vi "Handle.vi"(8 "error in (no error)":errorcluster, 10 "Zero Timeout Message Handler in":refnum<class "Zero Timeout Message Handler.lvclass">, 11 "Message in":refnum<class "Stop Msg.lvclass">) -> (0 "error out":errorcluster, 2 "Zero Timeout Message Handler out":refnum<class "Zero Timeout Message Handler.lvclass">)   [LabVIEW 2024, in "Zero Timeout Message Handler.lvlib" / "Stop Msg.lvclass"]
uses:
  Zero Timeout Message Handler/Zero Timeout Message Handler.lvclass
  Stop Msg.lvclass
  Stop Msg.lvclass/Stop Msg.ctl
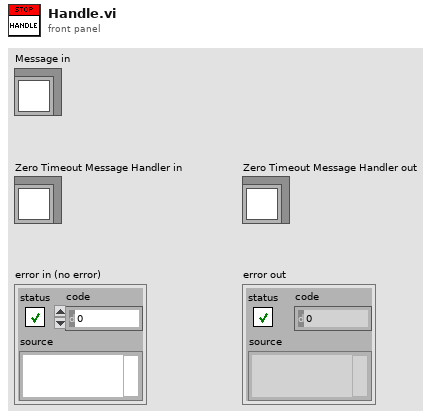
[diagram p1: front panel]
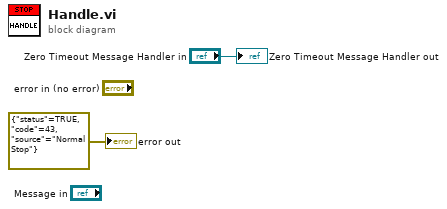
[diagram p0: block diagram]
diagram:
  "error out" <- errorcluster {"status"=TRUE, "code"=43, "source"="Normal Stop"} ("error out")
  "Zero Timeout Message Handler out" <- "Zero Timeout Message Handler in"
